vi "AlliGator Recompute Decay Statistics Histograms.vi"(7 "Decay Statistics Graph":refnum<vi>, 8 "Error In":errorcluster, 9 "Decay Statistics Bin":i32, 10 "Decays Min Values":sgl[](array[numeric]), 11 "Decays Max Values":sgl[](array[numeric])) -> (0 "Error Out":errorcluster)   [LabVIEW 2021, in "AlliGator Decay Statistics.lvlib"]
doc: "Rebins decay Min & Max histograms."
uses:
  AlliGator Decay Statistics.lvlib
  Histograms/Linear Histogram Options.ctl
  Histograms/Histogram Bin Option.ctl
  Histograms/Histogram Bin Position.ctl
  1f021b7e-425b-40a9-9546-7345520a62a8.vi
  b5ad749e-8322-46bf-8c18-040d7131fb1e.vi
  1f021b7e-425b-40a9-9546-7345520a62a8.vi/b1828c6e-eb0a-43e9-a724-8b596c52e435.vi
  1f021b7e-425b-40a9-9546-7345520a62a8.vi/7a6138ed-c001-4311-b538-9ba42ae7c7b1.vi
  1f021b7e-425b-40a9-9546-7345520a62a8.vi/52c6b4fa-501b-4af0-803b-8bab516ca5d3.vi
  1f021b7e-425b-40a9-9546-7345520a62a8.vi/d7237e10-35ab-4bcb-a0c6-4883c3f4c990.vi
  1f021b7e-425b-40a9-9546-7345520a62a8.vi/5fb5dd96-3b97-4592-ba56-58181c8e7105.vi
  1f021b7e-425b-40a9-9546-7345520a62a8.vi/8e13a849-a393-4484-9968-4af7b25c38d7.vi
  b5ad749e-8322-46bf-8c18-040d7131fb1e.vi/b1828c6e-eb0a-43e9-a724-8b596c52e435.vi
  b5ad749e-8322-46bf-8c18-040d7131fb1e.vi/7a6138ed-c001-4311-b538-9ba42ae7c7b1.vi
  b5ad749e-8322-46bf-8c18-040d7131fb1e.vi/52c6b4fa-501b-4af0-803b-8bab516ca5d3.vi
  b5ad749e-8322-46bf-8c18-040d7131fb1e.vi/d7237e10-35ab-4bcb-a0c6-4883c3f4c990.vi
  b5ad749e-8322-46bf-8c18-040d7131fb1e.vi/5fb5dd96-3b97-4592-ba56-58181c8e7105.vi
  b5ad749e-8322-46bf-8c18-040d7131fb1e.vi/8e13a849-a393-4484-9968-4af7b25c38d7.vi
  Time/High Resolution Timing.vi
  <userlib>/_OpenG.lib/array/array.llb/Filter 1D Array__ogtk.vi
  <userlib>/_OpenG.lib/array/array.llb/Filter 1D Array (SGL)__ogtk.vi
  <userlib>/_OpenG.lib/array/array.llb/Delete Elements from Array__ogtk.vi
  <userlib>/_OpenG.lib/array/array.llb/Delete Elements from 1D Array (DBL)__ogtk.vi
  <vilib>/Utility/error.llb/Error Cluster From Error Code.vi
  Graphs/XY Graph/XY Graph Add-Ons.lvlib
  Histograms/Histogram Window.lvlib
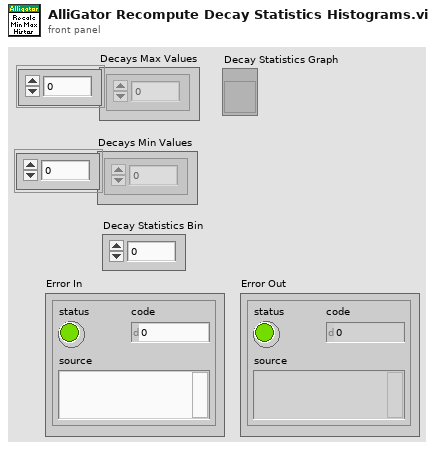
[diagram p1: front panel]
types:
  T1 = typedef "Histogram Window.lvlib/Linear Histogram Options.ctl" = cluster{"Bin Size":dbl, "Bin Number":i32, "Bin Option":T2, "Min Value":dbl, "Max Value":dbl, "Filter NaN & Infinite Values":bool, "Frequency Plot":bool, "Align Bins":bool, "Bin Location":T3, "Project Outside Values":bool, "Max Histogram Size":i32}
  T2 = typedef "Histogram Window.lvlib/Histogram Bin Option.ctl" = enum32{"Bin Number", "Bin Size"}
  T3 = typedef "Histogram Window.lvlib/Histogram Bin Position.ctl" = enum16{"Left", "Center", "Right"}
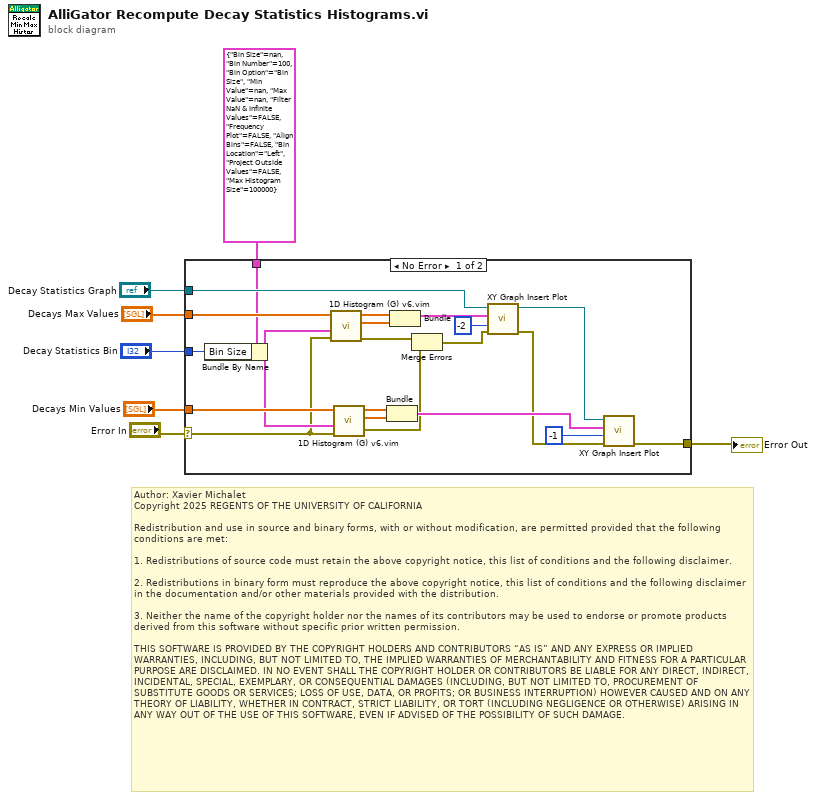
[diagram p0: block diagram]
diagram:
  # "Author: Xavier Michalet\nCopyright 2025 REGENTS OF THE UNIVERSITY OF CALIFORNIA\n\nRedistribution and use in source and binary forms, with or without modification, are permitted provided that the following conditions are met:\n\n1. Redistributions of source code must retain the above copyright notice, this list of conditions and the following disclaimer.\n\n2. Redistributions in binary form must reproduce the above copyright notice, this list of conditions and the following disclaimer in the documentation and/or other materials provided with the distribution.\n\n3. Neither the name of the copyright holder nor the names of its contributors may be used to endorse or promote products derived from this software without specific prior written permission.\n\nTHIS SOFTWARE IS PROVIDED BY THE COPYRIGHT HOLDERS AND CONTRIBUTORS “AS IS” AND ANY EXPRESS OR IMPLIED WARRANTIES, INCLUDING, BUT NOT LIMITED TO, THE IMPLIED WARRANTIES OF MERCHANTABILITY AND FITNESS FOR A PARTICULAR PURPOSE ARE DISCLAIMED. IN NO EVENT SHALL THE COPYRIGHT HOLDER OR CONTRIBUTORS BE LIABLE FOR ANY DIRECT, INDIRECT, INCIDENTAL, SPECIAL, EXEMPLARY, OR CONSEQUENTIAL DAMAGES (INCLUDING, BUT NOT LIMITED TO, PROCUREMENT OF SUBSTITUTE GOODS OR SERVICES; LOSS OF USE, DATA, OR PROFITS; OR BUSINESS INTERRUPTION) HOWEVER CAUSED AND ON ANY THEORY OF LIABILITY, WHETHER IN CONTRACT, STRICT LIABILITY, OR TORT (INCLUDING NEGLIGENCE OR OTHERWISE) ARISING IN ANY WAY OUT OF THE USE OF THIS SOFTWARE, EVEN IF ADVISED OF THE POSSIBILITY OF SUCH DAMAGE."
  n1 = case shown="No Error" "Error In" {
    selector: "Error In" -> [w10 w29]
    tunnel: "Decays Max Values" -> [w24 _]
    tunnel: "Decays Min Values" -> [w23 _]
    tunnel: "Decay Statistics Bin" -> [w13 _]
    tunnel: "Decay Statistics Graph" -> [w21 _]
    tunnel: [w15 w29] -> w2
    tunnel: T1 {"Bin Size"=nan, "Bin Number"=100, "Bin Option"=enum."Bin Size", "Min Value"=nan, "Max Value"=nan, "Filter NaN & Infinite Values"=FALSE, "Frequency Plot"=FALSE, "Align Bins"=FALSE, "Bin Location"=enum."Left", "Project Outside Values"=FALSE, "Max Histogram Size"=100000} ("Histogram Options") -> [w14 _]
    frame No Error {
      n2 = Bundle By Name(cluster=w14, "Bin Size"=w13) -> (w12:T1)
      n3 = call "1D Histogram (G) v6.vim"("Error In"=w10, "Histogram Options"=w12, "Array"=w24) -> ("Error Out"=w11:errorcluster, "Histogram"=w27:dbl[], "Axis"=w28:dbl[])  [unwired: 2 in, 4 out]
      n4 = call "1D Histogram (G) v6.vim"("Error In"=w10, "Histogram Options"=w12, "Array"=w23) -> ("Error Out"=w8:errorcluster, "Histogram"=w25:dbl[], "Axis"=w26:dbl[])  [unwired: 2 in, 4 out]
      n5 = Bundle("Axis"=w26, "Histogram"=w25) -> (w19:cluster{"Axis":dbl[], "Histogram":dbl[]})  [unwired: 1 in]
      n6 = Bundle("Axis"=w28, "Histogram"=w27) -> (w22:cluster{"Axis":dbl[], "Histogram":dbl[]})  [unwired: 1 in]
      n7 = Merge Errors(w11, w8) -> (w9:errorcluster)
      n8 = call "XY Graph Insert Plot.vi"("Error In"=w9, "Plot Index (Default Inf: Append to End)"=-2, "New Plot"=w22, "Multiplot XY Graph Refnum in"=w21) -> ("Error Out"=w17:errorcluster, "Multiplot XY Graph Refnum out"=w18:refnum<vi>)  [unwired: 5 in, 1 out]
      n9 = call "XY Graph Insert Plot.vi"("Error In"=w17, "Plot Index (Default Inf: Append to End)"=-1, "New Plot"=w19, "Multiplot XY Graph Refnum in"=w18) -> ("Error Out"=w15:errorcluster)  [unwired: 5 in, 2 out]
    }
    frame Error {
    }
  }
  "Error Out" <- w2
